vi "Update Offset of Disabled Sites.vi"(5 "Enabled Sites":i32[](array[numeric]), 7 "Calibration Cfg File":T2={"Path"=path "C:/Users/Public/Documents/National Instruments/Golden Units Calibration Tool/Calibration Config/Golden Units Calibration.csv", "Config Data"=[{"Section Name"="General", "Section Data"=[["Match_SeqFile", "Golden Units Calibration.seq"], ["CorrOffsetFilePath", "C:\\Users\\Public\\Documents\\National Instruments\\TestStand 2019 (64-bit)\\Examples\\Golden Units Calibration Tool\\Supporting Materials\\Golden Units\\Offset.txt"]]}, {"Section Name"="PluginCfg", "Section Data"=[["GUCalibration.lvlib", "Enabled:TRUE;Trigger:TRUE;Option:TRUE;Limit:TRUE;Offset:TRUE;Report:TRUE"]]}, {"Section Name"="PluginSpecific", "Section Data"=[["CorrOffsetFilePath", "C:\\Users\\Public\\Documents\\National Instruments\\TestStand 2019 (64-bit)\\Examples\\Golden Units Calibration Tool\\Supporting Materials\\Golden Units\\Offset.txt"], ["GUBenchFilePath", "C:\\Users\\Public\\Documents\\National Instruments\\TestStand 2019 (64-bit)\\Examples\\Golden Units Calibration Tool\\Supporting Materials\\Golden Units\\GU_Bench.csv"], ["CalType", "0"], ["CalibrationEnd", "FALSE"], ["CalCheckPass", "TRUE"], ["IsCalibration", "TRUE"], ["Enabled_Sites", "0;1"], ["GU_Selected", "1;3"], ["GU_Arrange", "1_3;3_1"], ["GU_Test_Count", "3_3;3_3"], ["Curr_GU", ""], ["Curr_GU_Index", "2"], ["Curr_GU_Test_Count", ""], ["Loop_Count_Per_Batch", "3"], ["Curr_GU_Target_Count", ""], ["All_Available_GU", "1;2;3"], ["GU_Test_Result", "111_111;111_111"], ["Curr_GU_Test_Result", ""], ["GU_Iteration_Done", "TRUE"]]}, {"Section Name"="CalCfg", "Section Data"=[["Index", "TestName", "TestNumber", "Units", "ENABLE_CALIBRATION", "ENABLE_CHECK", "GU_CAL_LLIM", "GU_CAL_HLIM", "GU_CHECK_LLIM", "GU_CHECK_HLIM", "GU1", "GU2", "GU3"], ["1", "TXP - Average Mean Power", "1001", "dBm", "1", "1", "-3", "3", "-1", "1", "-11.5", "-12.8", "-12.3"], ["2", "TXP - Peak to Average Ratio", "1002", "dB", "1", "1", "-3", "3", "-1", "1", "9.6", "10.1", "10.2"], ["3", "TXP - Maximum Power", "1003", "dBm", "1", "1", "-3", "3", "-1", "1", "-2.5", "-1.8", "-2.1"], ["4", "TXP - Minimum Power", "1004", "dBm", "0", "0", "0", "0", "0", "0", "0", "0", "0"], ["5", "AMPM - Mean RMS EVM", "2001", "%", "1", "1", "-0.25", "0.25", "-0.1", "0.1", "0.15", "0.21", "0.23"], ["6", "AMPM - Mean Linear Gain", "2002", "dB", "1", "1", "-1.5", "1.5", "-1", "1", "-2.8", "-3.5", "-2.9"]]}]}, 8 "error in":errorcluster, 11 "CorrOffset File In":T1={"File Path"=path "C:/Users/Public/Documents/National Instruments/TestStand 2019 (64-bit)/Examples/Golden Units Calibration Tool/Supporting Materials/Golden Units/Offset.txt", "Backup File Path"=path "", "Offset Data"=[{"Section Name"="!--CalTime0=20210830141642,CalTime1=20210830141642,CalTime2=20210830134752,CalTime3=20210830141832--/", "Section Data"=[]}, {"Section Name"="SemiconductorModuleTests", "Section Data"=[["<SequenceName>", "<StepName>", "<StepId>", "<TestNumber>", "<Site_0_Offset>", "<Site_1_Offset>", "<Site_2_Offset>", "<Site_3_Offset>"], ["MainSequence", "Simulate SpecAn TXP Test", "ID#:RNoVwgHm6xG7pwAMKVCzqC", "1001", "8.000000E-1", "2.000000E-1", "6.000000E-1", "1.000000E-1"], ["MainSequence", "Simulate SpecAn TXP Test", "ID#:RNoVwgHm6xG7pwAMKVCzqC", "1002", "-8.000000E-1", "-2.000000E-1", "-6.000000E-1", "-1.000000E-1"], ["MainSequence", "Simulate SpecAn TXP Test", "ID#:RNoVwgHm6xG7pwAMKVCzqC", "1003", "-2.400000E+0", "-6.000000E-1", "-1.800000E+0", "-3.000000E-1"], ["MainSequence", "Simulate SpecAn TXP Test", "ID#:RNoVwgHm6xG7pwAMKVCzqC", "1004", "0.000000E+0", "0.000000E+0", "0.000000E+0", "0.000000E+0"], ["MainSequence", "Simulate SpecAn AMPM Test", "ID#:MlU3iQfm6xG7pwAMKVCzqC", "2001", "-8.000000E-2", "-2.000000E-2", "-6.000000E-2", "-1.000000E-2"], ["MainSequence", "Simulate SpecAn AMPM Test", "ID#:MlU3iQfm6xG7pwAMKVCzqC", "2002", "1.200000E+0", "3.000000E-1", "9.000000E-1", "1.500000E-1"]]}, {"Section Name"="/SemiconductorModuleTests", "Section Data"=[]}]}) -> (0 "error out":errorcluster, 1 "Update OK":bool, 3 "CorrOffset File Out":T1={"File Path"=path "C:/Users/Public/Documents/National Instruments/TestStand 2019 (64-bit)/Examples/Golden Units Calibration Tool/Supporting Materials/Golden Units/Offset.txt", "Backup File Path"=path "", "Offset Data"=[{"Section Name"="!--CalTime0=20210830141642,CalTime1=20210830141642,CalTime2=20210830134752,CalTime3=20210830141832--/", "Section Data"=[]}, {"Section Name"="SemiconductorModuleTests", "Section Data"=[["<SequenceName>", "<StepName>", "<StepId>", "<TestNumber>", "<Site_0_Offset>", "<Site_1_Offset>", "<Site_2_Offset>", "<Site_3_Offset>"], ["MainSequence", "Simulate SpecAn TXP Test", "ID#:RNoVwgHm6xG7pwAMKVCzqC", "1001", "8.000000E-1", "2.000000E-1", "6.000000E-1", "1.000000E-1"], ["MainSequence", "Simulate SpecAn TXP Test", "ID#:RNoVwgHm6xG7pwAMKVCzqC", "1002", "-8.000000E-1", "-2.000000E-1", "-6.000000E-1", "-1.000000E-1"], ["MainSequence", "Simulate SpecAn TXP Test", "ID#:RNoVwgHm6xG7pwAMKVCzqC", "1003", "-2.400000E+0", "-6.000000E-1", "-1.800000E+0", "-3.000000E-1"], ["MainSequence", "Simulate SpecAn TXP Test", "ID#:RNoVwgHm6xG7pwAMKVCzqC", "1004", "0.000000E+0", "0.000000E+0", "0.000000E+0", "0.000000E+0"], ["MainSequence", "Simulate SpecAn AMPM Test", "ID#:MlU3iQfm6xG7pwAMKVCzqC", "2001", "-8.000000E-2", "-2.000000E-2", "-6.000000E-2", "-1.000000E-2"], ["MainSequence", "Simulate SpecAn AMPM Test", "ID#:MlU3iQfm6xG7pwAMKVCzqC", "2002", "1.200000E+0", "3.000000E-1", "9.000000E-1", "1.500000E-1"]]}, {"Section Name"="/SemiconductorModuleTests", "Section Data"=[]}]})   [LabVIEW 2020, in "GUCalibration2.lvlib"]
uses:
  GUCalibration2.lvlib
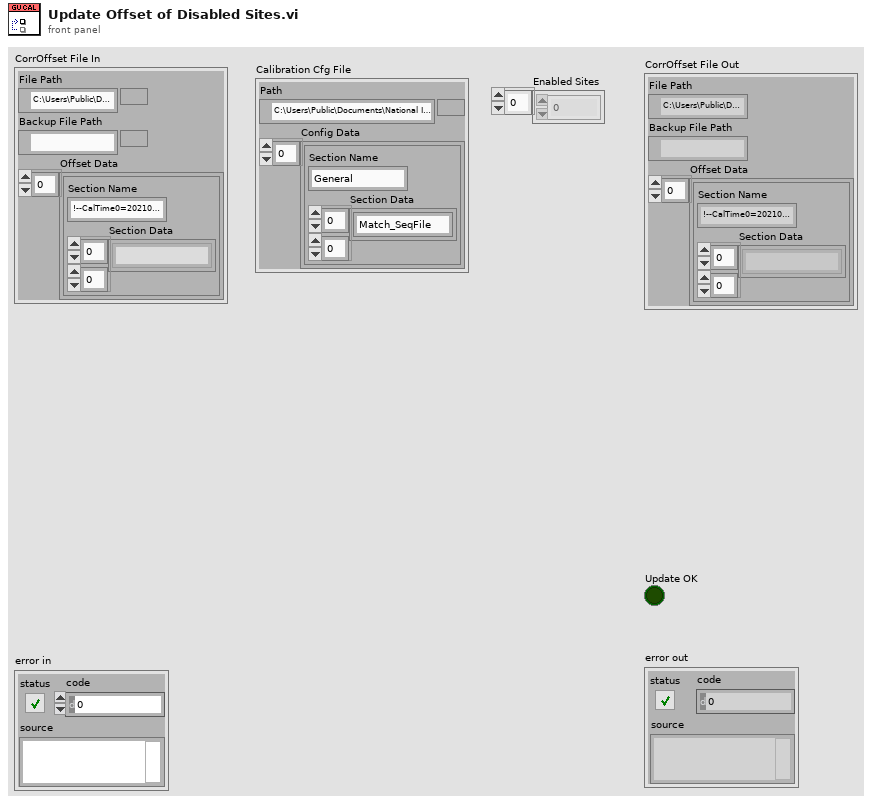
[diagram p1: front panel]
types:
  T1 = cluster{"File Path":path, "Backup File Path":path, "Offset Data":cluster{"Section Name":string, "Section Data":string[][]}[]}
  T2 = cluster{"Path":path, "Config Data":cluster{"Section Name":string, "Section Data":string[][]}[]}
  T3 = cluster{"Section Name":string, "Section Data":string[][]}[]
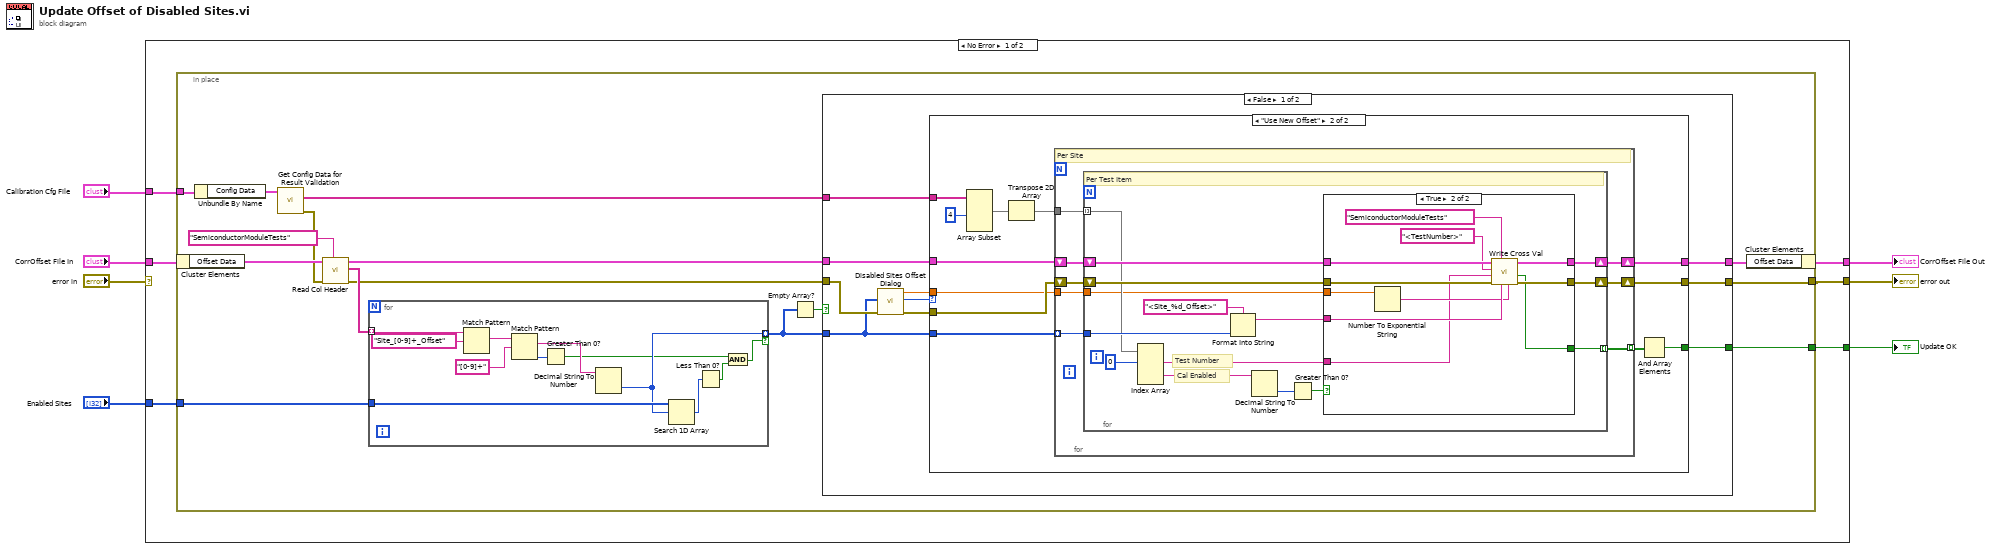
[diagram p0: block diagram]
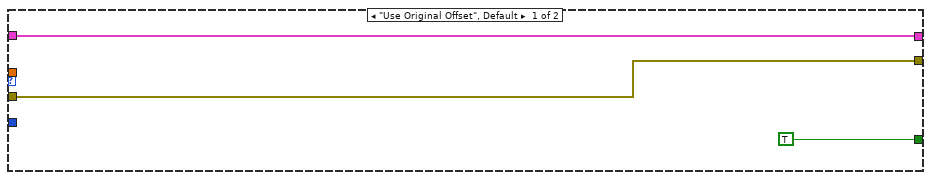
[diagram p2: hidden frame]
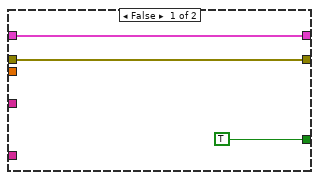
[diagram p3: hidden frame]
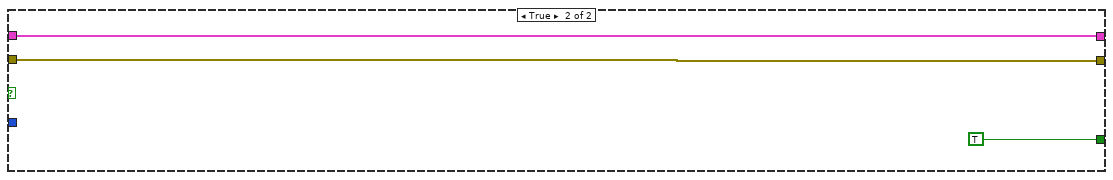
[diagram p4: hidden frame]
diagram:
  n1 = case shown="No Error" "error in" {
    selector: "error in" -> [_ w106]
    tunnel: "CorrOffset File In" -> [w13 w107]
    tunnel: [w12 w107] -> w3
    tunnel: [w10 w106] -> w7
    tunnel: [w11 _] -> w6
    tunnel: "Enabled Sites" -> [w9 _]
    tunnel: "Calibration Cfg File" -> [w8 _]
    frame No Error {
      n2 = in-place {
        in-place-border: [w27] -> w10
        in-place-border: [w26] -> w11
        in-place-border: w9 -> [w21]
        in-place-border: w8 -> [w20]
        n3 = in-place-cluster #1(w13) -> ("Offset Data"=w25:T3)
        n4 = Unbundle By Name(w20) -> ("Config Data"=w19:T3)
        n5 = call "Get Config Data for Result Validation.vi"("Config Data"=w19) -> ("error out"=w17:errorcluster, "Config Data"=w18:string[][])  [unwired: 6 in, 3 out]
        n6 = call "Read Col Header.vi"("Section Name"="SemiconductorModuleTests", "error in (no error)"=w17, "Config Data"=w25) -> ("error out"=w16:errorcluster, "Column Header"=w22:string[], "Config Data dup"=w23:T3)  [unwired: 4 in, 2 out]
        n7 = for {
          tunnel: w22 -> [w105] mode=indexing
          tunnel: [w98] -> w15 mode=indexing if=w94
          tunnel: w21 -> [w99]
          n8 = Match Pattern(string=w105, regular expression="Site_[0-9]+_Offset") -> (match substring=w103:string)  [unwired: 1 in, 3 out]
          n9 = Match Pattern(string=w103, regular expression="[0-9]+") -> (match substring=w100:string, offset past match=w101:i32)  [unwired: 1 in, 2 out]
          n10 = Greater Than 0?(x=w101) -> (x > 0?=w96:bool)
          n11 = Decimal String To Number(string=w100) -> (number=w98:i32)  [unwired: 2 in, 1 out]
          n12 = Search 1D Array(1D array=w99, element=w98) -> (index of element=w97:i32)  [unwired: 1 in]
          n13 = Less Than 0?(x=w97) -> (x < 0?=w95:bool)
          n14 = And(x=w96, y=w95) -> (x .and. y?=w94:bool)
        }
        n15 = Empty Array?(array=w15) -> (empty?=w14:bool)
        n16 = case shown="False" w14 {
          tunnel: [w38 w93] -> w28
          tunnel: [w37 w92] -> w27
          tunnel: [w36 TRUE] -> w26
          tunnel: w23 -> [w35 w93]
          tunnel: w18 -> [w34 _]
          tunnel: w16 -> [w33 w92]
          tunnel: w15 -> [w29 _]
          frame False {
            n17 = call "Disabled Sites Offset Dialog.vi"("error in"=w33, "Disabled Sites"=w29) -> ("error out"=w32:errorcluster, "Offset Update Option Out"=w30:enum32{"Use Original Offset", "Use New Offset"}, "New Offset  Out"=w31:dbl)  [unwired: 7 in]
            n18 = case shown="\"Use New Offset\"" w30 {
              tunnel: [w41 w53] -> w38
              tunnel: [w40 w52] -> w37
              tunnel: [TRUE w51] -> w36
              tunnel: w35 -> [w41 w50]
              tunnel: w34 -> [_ w49]
              tunnel: w29 -> [_ w46]
              tunnel: w32 -> [w40 w44]
              tunnel: w31 -> [_ w43]
              frame "Use Original Offset", Default {
              }
              frame "Use New Offset" {
                n19 = Array Subset(array=w49, length (row)=4 ("length")) -> (w45:string[][])  [unwired: 3 in]
                n20 = Transpose 2D Array(2D array=w45) -> (transposed array=w42:string[][])
                n21 = for {
                  shift-right: [w59] -> w53
                  shift-left: w50 -> [w61]
                  shift-right: [w58] -> w52
                  shift-left: w44 -> [w60]
                  tunnel: [w57] -> w47 mode=indexing
                  tunnel: w46 -> [w56] mode=indexing
                  tunnel: w42 -> [w55]
                  tunnel: w43 -> [w54]
                  # "Per Site"
                  n22 = for {
                    tunnel: [w71] -> w57 mode=indexing
                    shift-right: [w72] -> w58
                    shift-left: w60 -> [w75]
                    shift-right: [w73] -> w59
                    shift-left: w61 -> [w76]
                    tunnel: w56 -> [w69]
                    tunnel: w55 -> [w68] mode=indexing
                    tunnel: w54 -> [w63]
                    # "Cal Enabled"
                    # "Test Number"
                    # "Per Test Item"
                    n23 = Index Array(array=w68, index #1=0 ("index")) -> (element #1=w66:string, element #3=w65:string)  [unwired: 3 in, 2 out]
                    n24 = Format Into String(format string="<Site_%d_Offset>", w69) -> (resulting string=w74:string)  [unwired: 2 in, 1 out]
                    n25 = Decimal String To Number(string=w65) -> (number=w64:i32)  [unwired: 2 in, 1 out]
                    n26 = Greater Than 0?(x=w64) -> (x > 0?=w62:bool)
                    n27 = case shown="True" w62 {
                      tunnel: w76 -> [w79 w90]
                      tunnel: w75 -> [w78 w89]
                      tunnel: w74 -> [_ w86]
                      tunnel: [w79 w85] -> w73
                      tunnel: [w78 w84] -> w72
                      tunnel: [TRUE ("Find?") w83] -> w71
                      tunnel: w66 -> [_ w81]
                      tunnel: w63 -> [_ w80]
                      frame False {
                      }
                      frame True {
                        n28 = Number To Exponential String(number=w80) -> (E-format string=w82:string)  [unwired: 3 in]
                        n29 = call "Write Cross Val.vi"("Col Header Val 2"=w82, "Col Header Name 2"=w86, "Section Name"="SemiconductorModuleTests", "error in (no error)"=w89, "Col Header Val 1"=w81, "Col Header Name 1"="<TestNumber>", "Config Data"=w90) -> ("error out"=w84:errorcluster, "Find?"=w83:bool, "Config Data dup"=w85:T3)  [unwired: 2 in]
                      }
                    }
                  }
                }
                n30 = And Array Elements(Boolean array=w47) -> (logical AND=w51:bool)
              }
            }
          }
          frame True {
          }
        }
        n31 = in-place-cluster #1("Offset Data"=w28) -> (w12:T1)
      }
    }
    frame Error {
    }
  }
  "error out" <- w7
  "Update OK" <- w6
  "CorrOffset File Out" <- w3
